vi "Tester Auto-Refresh.vi"() -> ()   [LabVIEW 2014, in "CAP-USB-1.lvlib"]
uses:
  CAP-USB-1.lvlib
  DriverMasterSync/build/DriverMasterSync.lvlibp/APIs/Data Queue/Acquisition Data 1 Sample Cluster.ctl
  CAP-USB-1Class/CAP-USB-1.lvclass
  DriverMasterSync/build/DriverMasterSync.lvlibp/APIs/Data Queue/WINFAS 2 Data Queue.lvlib
panel:
  out "Numeric":i32
  out "error out":errorcluster
  in  "stop":bool
  out "1 Sample":T1
  in  "Leer":bool
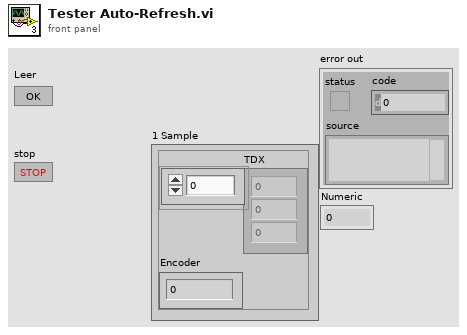
[diagram p1: front panel]
types:
  T1 = typedef "DriverMasterSync.lvlibp/WINFAS 2 Data Queue.lvlib/Acquisition Data 1 Sample Cluster.ctl" = cluster{"TDX":sgl[], "Encoder":sgl}
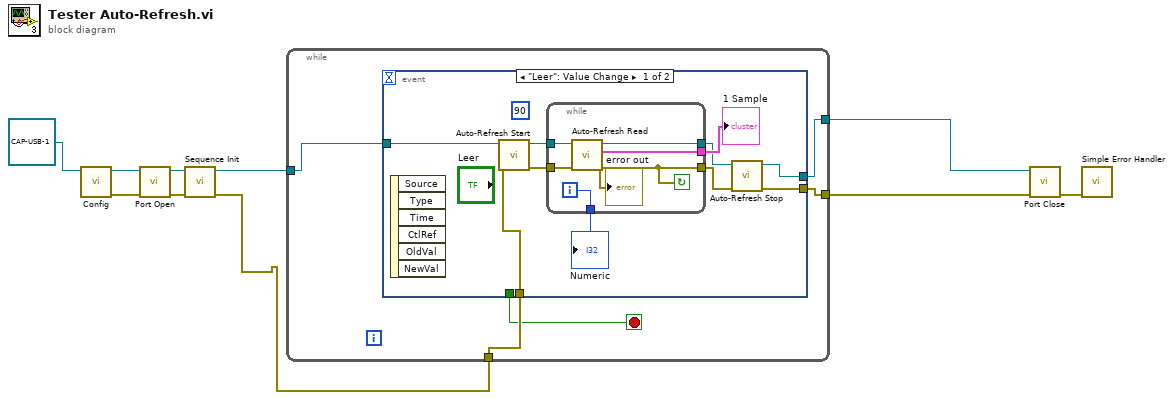
[diagram p0: block diagram]
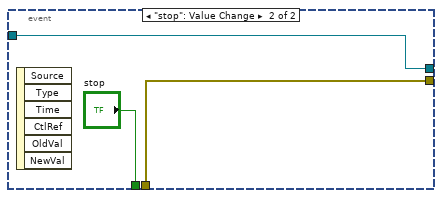
[diagram p2: hidden frame]
diagram:
  n1 = call-dynamic "Config.vi"("CAP-USB-1 in"=refnum<class "CAP-USB-1.lvclass"> refnum) -> ("error out"=w10:errorcluster, "CAP-USB-1 out"=w8:refnum<class "CAP-USB-1.lvclass">)  [unwired: 8 in, 1 out]
  n2 = call-dynamic "Port Open.vi"("error in (no error)"=w10, "CAP-USB-1 in"=w8) -> ("error out"=w6:errorcluster, "CAP-USB-1 out"=w7:refnum<class "CAP-USB-1.lvclass">)  [unwired: 8 in]
  n3 = call-dynamic "Sequence Init.vi"("error in (no error)"=w6, "CAP-USB-1 in"=w7) -> ("error out"=w3:errorcluster, "CAP-USB-1 out"=w4:refnum<class "CAP-USB-1.lvclass">)  [unwired: 8 in]
  n4 = while {
    tunnel: w4 -> [w15]
    tunnel: w3 -> [w14]
    tunnel: [w13] -> w2
    tunnel: [w12] -> w1
    stop <- w11 stop-if-true
    n5 = event shown="[0] \"Leer\": Value Change" {
      selector: _ -> [_ _]
      dyn-events: _ -> [_ _]
      timeout: _ -> [_ _]
      tunnel: w15 -> [w19 w33]
      tunnel: w14 -> [w18 w32]
      tunnel: [w21 w33] -> w13
      tunnel: [w22 w32] -> w12
      tunnel: [_ "stop"] -> w11
      event "Leer": Value Change {
        (unwired) 90
        n6 = event-data() -> ()  [unwired: 1 in, 6 out]
        n7 = call-dynamic "Auto-Refresh Start.vi"("error in (no error)"=w18, "CAP-USB-1 in"=w19) -> ("error out"=w17:errorcluster, "CAP-USB-1 out"=w20:refnum<class "CAP-USB-1.lvclass">)  [unwired: 8 in]
        n8 = while {
          tunnel: [w31] -> w25
          tunnel: w20 -> [w29]
          tunnel: [w30] -> w24
          tunnel: w17 -> [w28]
          tunnel: [w27] -> w23
          tunnel: [w26] -> w16
          i -> [w26]
          stop <- w27 continue-if-true
          n9 = call-dynamic "Auto-Refresh Read.vi"("error in (no error)"=w28, "CAP-USB-1 in"=w29) -> ("error out"=w27:errorcluster, "1 Sample"=w31:T1, "CAP-USB-1 out"=w30:refnum<class "CAP-USB-1.lvclass">)  [unwired: 6 in, 1 out]
          "error out" <- w27
        }
        "1 Sample" <- w25
        "Numeric" <- w16
        n10 = call-dynamic "Auto-Refresh Stop.vi"("error in (no error)"=w23, "CAP-USB-1 in"=w24) -> ("error out"=w22:errorcluster, "CAP-USB-1 out"=w21:refnum<class "CAP-USB-1.lvclass">)  [unwired: 8 in]
      }
      event "stop": Value Change {
        n11 = event-data() -> ()  [unwired: 1 in, 6 out]
      }
    }
  }
  n12 = call-dynamic "Port Close.vi"("error in (no error)"=w1, "CAP-USB-1 in"=w2) -> ("error out"=w5:errorcluster)  [unwired: 8 in, 1 out]
  n13 = call <vilib>:"Simple Error Handler.vi"("error in (no error)"=w5) -> ()  [unwired: 4 in, 5 out]
